vi "Notify Subscribers.vi"(8 "error in (no error)":errorcluster, 10 "PublishRequest":refnum<class "PublishRequest.lvclass">, 11 "Topic in":refnum<class "Topic.lvclass">) -> (0 "error out":errorcluster, 3 "Topic out":refnum<class "Topic.lvclass">)   [LabVIEW 2017, in "Mediator.lvlib" / "Topic.lvclass"]
doc: "<License>\nCopyright © 2017 Composed Systems, LLC | All rights reserved\nwww.composed.io\n\nAuthor: Ethan Stern <ethan.stern@composed.io>\n\nThis software is provided \"AS IS\" WITHOUT WARRANTIES, either express or implied, AND IS FOR EDUCATIONAL PURPOSES ONLY.\n</License>"
uses:
  Topic.lvclass
  IMediator/PublishRequest/PublishRequest.lvclass
  Topic.lvclass/Topic.ctl
  IMediator/PublishRequest/PublishRequest.lvclass/PublishRequest.ctl
  IMediator/ISubscriptionPolicy/ISubscriptionPolicy.lvclass/ISubscriptionPolicy.ctl
  IMediator/ISubscriptionPolicy/Execute Subscription Policy.vi
  IMediator/ISubscriptionPolicy/ISubscriptionPolicy.lvclass
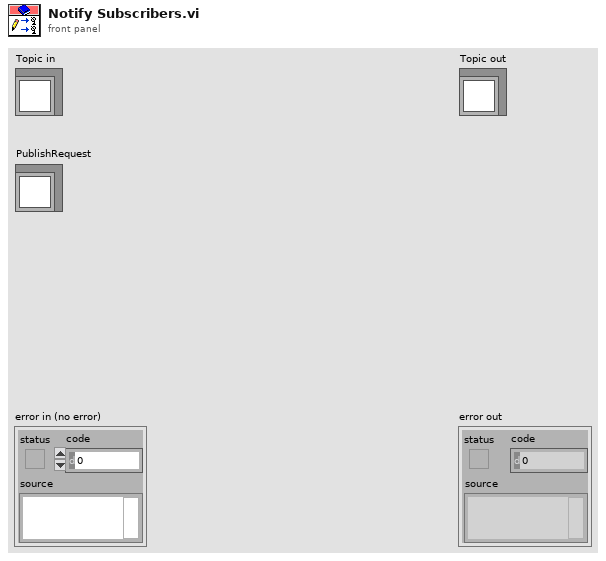
[diagram p1: front panel]
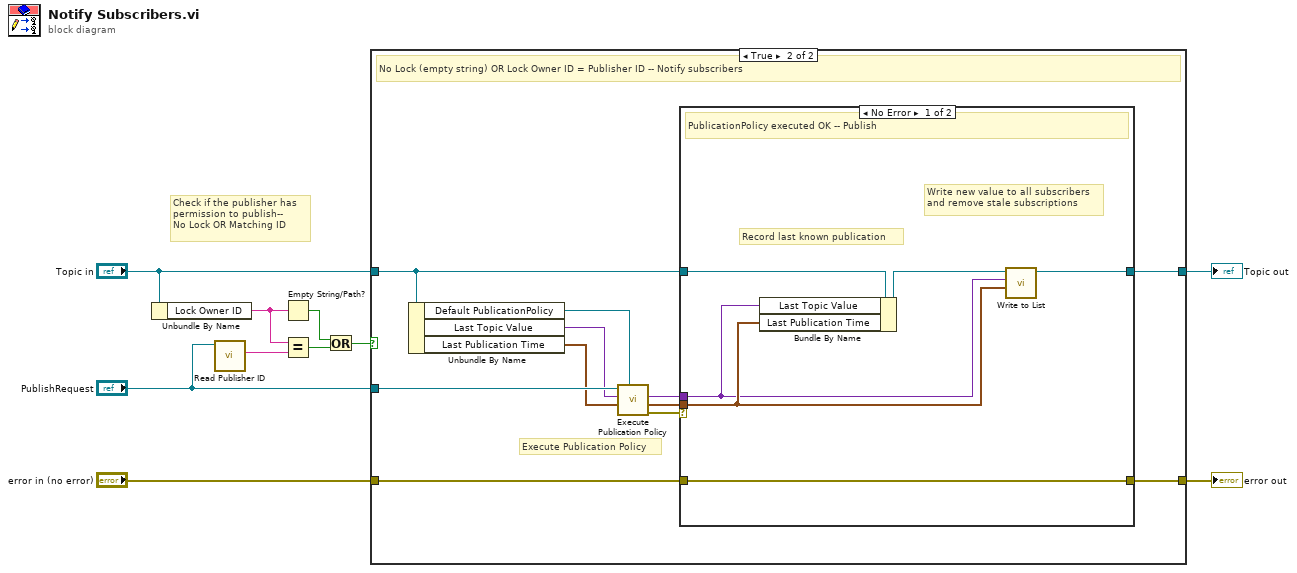
[diagram p0: block diagram]
diagram:
  # "Check if the publisher has\npermission to publish--\nNo Lock OR Matching ID"
  n1 = Unbundle By Name("Topic in") -> ("Lock Owner ID"=w6:string)
  n2 = call "Read Publisher ID.vi"("PublishRequest In"="PublishRequest") -> ("Publisher ID"=w1:string)  [unwired: 10 in]
  n3 = Empty String/Path?(string/path=w6) -> (empty?=w5:bool)
  n4 = Equal?(x=w6, y=w1) -> (x = y?=w4:bool)
  n5 = Or(x=w5, y=w4) -> (x .or. y?=w3:bool)
  n6 = case shown="True" w3 {
    tunnel: "error in (no error)" -> [w12 w23]
    tunnel: [w12 w22] -> w9
    tunnel: [w11 w21] -> w8
    tunnel: "Topic in" -> [w11 w19]
    tunnel: "PublishRequest" -> [_ w20]
    frame False {
      # "This publication was not from the lock holder -- Ignore it"
    }
    frame True {
      # "Execute Publication Policy"
      # "No Lock (empty string) OR Lock Owner ID = Publisher ID -- Notify subscribers"
      n7 = Unbundle By Name(w19) -> ("Default PublicationPolicy"=w18:refnum<class "IPublicationPolicy.lvclass">, "Last Topic Value"=w17:variant, "Last Publication Time"=w16:timestamp)
      n8 = call-dynamic "Execute Publication Policy.vi"("Default PublicationPolicy"=w18, "Last Publish Time"=w16, "Last Published Value"=w17, "PublishRequest"=w20) -> ("error out (Reject Publication)"=w14:errorcluster, "Publication Time"=w13:timestamp, "Value to Publish"=w15:variant)  [unwired: 5 in]
      n9 = case shown="No Error" w14 {
        tunnel: w23 -> [w29 w31]
        tunnel: [w29 w31] -> w22
        tunnel: [w28 w30] -> w21
        tunnel: w19 -> [w26 w30]
        tunnel: w15 -> [w24 _]
        tunnel: w13 -> [w25 _]
        frame No Error {
          # "Write new value to all subscribers\nand remove stale subscriptions"
          # "Record last known publication"
          # "PublicationPolicy executed OK -- Publish"
          n10 = Bundle By Name(cluster=w26, "Last Topic Value"=w24, "Last Publication Time"=w25) -> (w27:refnum<class "Topic.lvclass">)
          n11 = call "Write to List.vi"("Publication Time"=w25, "Value to Publish"=w24, "Topic in"=w27) -> ("Topic out"=w28:refnum<class "Topic.lvclass">)  [unwired: 8 in]
        }
        frame Error {
          # "Error executing PublicationPolicy -- Do not publish"
        }
      }
    }
  }
  "error out" <- w9
  "Topic out" <- w8
